vi "Read Menu Button Visible.vi"(9 "IOName in":refnum<class "IOName.lvclass">) -> (3 "IOName out":refnum<class "IOName.lvclass">, 4 "Menu Button Visible":bool)   [LabVIEW 2014, in "IOName.lvclass"]
uses:
  IOName.lvclass
  IOName.lvclass/IOName.ctl
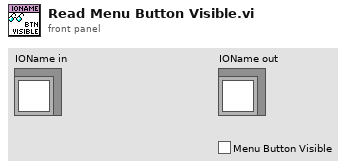
[diagram p1: front panel]
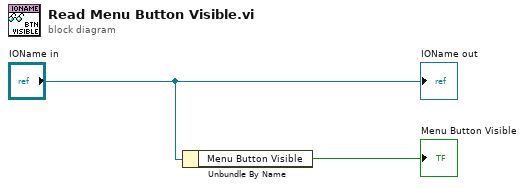
[diagram p0: block diagram]
diagram:
  n1 = Unbundle By Name("IOName in") -> ("Menu Button Visible"=→"Menu Button Visible":bool)
  "IOName out" <- "IOName in"
